vi "SearchForTwoInLine.vi"(5 "NumericGameboard":i8[](array[numeric])) -> (1 "Blocking Indices":i8[](array[numeric]), 2 "Wining Indices":i8[](array[numeric]))   [LabVIEW 2020]
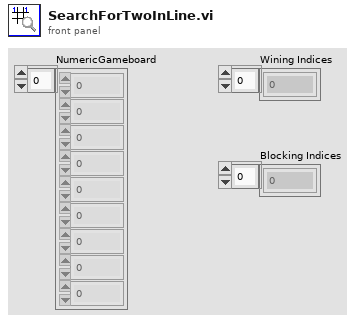
[diagram p1: front panel]
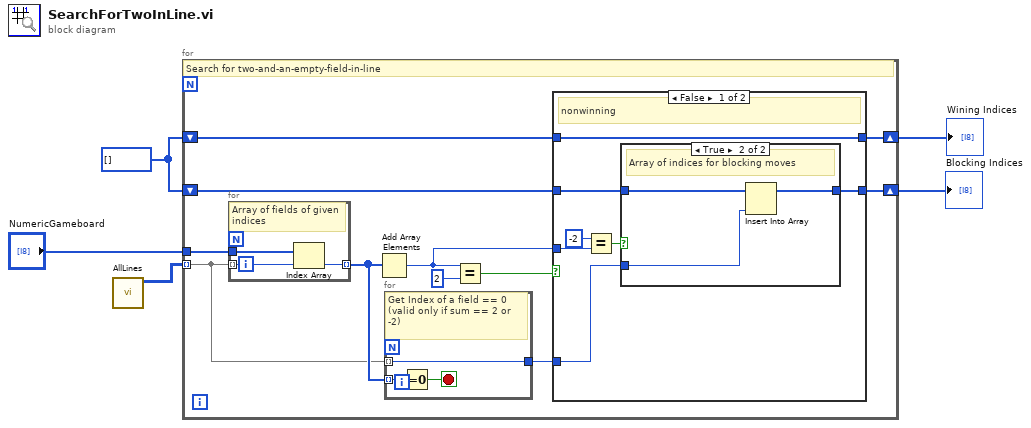
[diagram p0: block diagram]
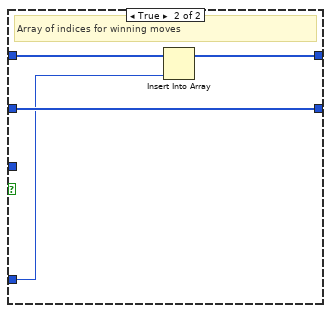
[diagram p3: hidden frame]
diagram:
  w5 = i8[] []
  n1 = call "AllLines.vi"() -> ("Lines"=w1:i8[][])  [unwired: 11 in]
  n2 = for {
    tunnel: w1 -> [w8] mode=indexing
    tunnel: "NumericGameboard" -> [w16]
    shift-right: [w13] -> w3
    shift-left: w5 -> [w12]
    shift-right: [w10] -> w2
    shift-left: w5 -> [w11]
    # "Search for two-and-an-empty-field-in-line"
    n3 = for {
      tunnel: w8 -> [w36] mode=indexing
      tunnel: w16 -> [w37]
      tunnel: [w35] -> w9 mode=indexing
      # "Array of fields of given indices"
      n4 = Index Array(array=w37, index=w36) -> (element=w35:i8)
    }
    n5 = Add Array Elements(numeric array=w9) -> (sum=w6:i8)
    n6 = for {
      tunnel: w9 -> [w19] mode=indexing
      tunnel: w8 -> [w17] mode=indexing
      tunnel: [w17] -> w7
      stop <- w18 stop-if-true
      # "Get Index of a field == 0\n(valid only if sum == 2 or -2)"
      n7 = Equal To 0?(x=w19) -> (x = 0?=w18:bool)
    }
    n8 = Equal?(x=w6, y=i8 2) -> (x = y?=w14:bool)
    n9 = case shown="False" w14 {
      tunnel: [w22 w34] -> w13
      tunnel: w12 -> [w23 w34]
      tunnel: w11 -> [w20 w33]
      tunnel: [w20 w32] -> w10
      tunnel: w7 -> [w21 w31]
      tunnel: w6 -> [w25 _]
      frame False {
        # "nonwinning"
        n10 = Equal?(x=i8 -2, y=w25) -> (x = y?=w26:bool)
        n11 = case shown="True" w26 {
          tunnel: w23 -> [w27 w30]
          tunnel: [w27 w29] -> w22
          tunnel: w21 -> [_ w28]
          frame False {
          }
          frame True {
            # "Array of indices for blocking moves"
            n12 = Insert Into Array(array=w30, new element=w28) -> (w29:i8[])  [unwired: 1 in]
          }
        }
      }
      frame True {
        # "Array of indices for winning moves"
        n13 = Insert Into Array(array=w33, new element=w31) -> (w32:i8[])  [unwired: 1 in]
      }
    }
  }
  "Blocking Indices" <- w3
  "Wining Indices" <- w2
